vi "Determine Chassis State.vi"(5 "Allowable Variation from Idea":dbl, 7 "Ideal Lateral Slip":dbl, 9 "Steering Angle":dbl, 10 "Chassis Speed":dbl, 11 "Chassis Yaw Rate":dbl) -> (1 "Lateral Slip":bool, 2 "Error":dbl)   [LabVIEW 2015]
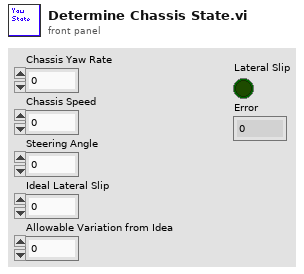
[diagram p1: front panel]
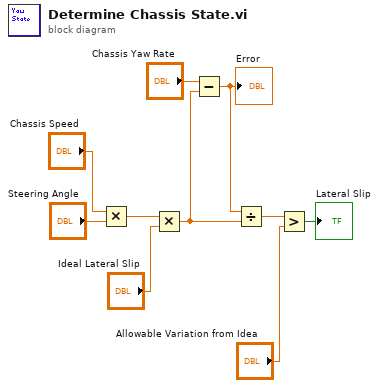
[diagram p0: block diagram]
diagram:
  n1 = Multiply(x="Chassis Speed", y="Steering Angle") -> (x*y=w8:dbl)
  n2 = Multiply(x=w8, y="Ideal Lateral Slip") -> (x*y=w5:dbl)
  n3 = Subtract(x="Chassis Yaw Rate", y=w5) -> (x-y=w1:dbl)
  "Error" <- w1
  n4 = Divide(x=w1, y=w5) -> (x/y=w4:dbl)
  n5 = Greater?(x=w4, y="Allowable Variation from Idea") -> (0:→"Lateral Slip":bool)
